vi "Configure Edge Trigger.vi"(6 "HF Rejection":bool=TRUE, 7 "Level":dbl, 8 "error in (no error)":errorcluster, 9 "Slope":u16(ring) items=["Rising", "Falling"], 10 "Function":u16(ring) items=["Voltage: DC", "Voltage: AC", "Current: DC", "Current: AC", "2W Resistance", "4W Resistance", "Diode", "Capacitance", "Temperature", "Continuity", "Frequency", "Period", "Ratio", "Digitize Voltage", "Digitize Current"], 11 "VISA resource name":refnum<visa-resource-name>) -> (0 "error out":errorcluster, 3 "VISA resource name out":refnum<visa-resource-name>)   [LabVIEW 2021, in "Keithley DMM7510.lvlib"]
doc: "This VI sets the slope and level of the analog edge trigger. This also enables or disables the high frequency rejection for analog trigger."
uses:
  Keithley DMM7510.lvlib
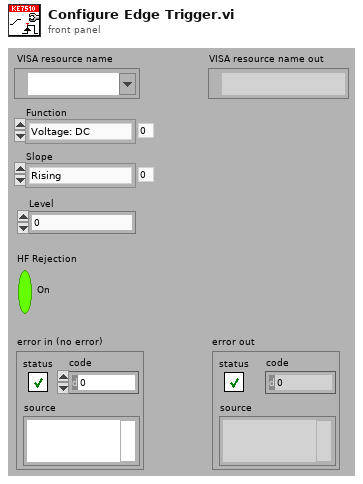
[diagram p1: front panel]
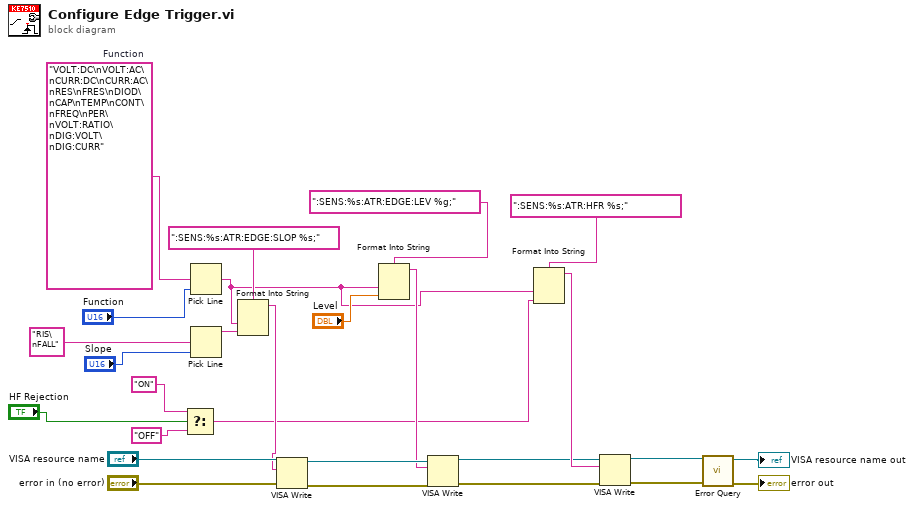
[diagram p0: block diagram]
diagram:
  w23 = "VOLT:DC\nVOLT:AC\nCURR:DC\nCURR:AC\nRES\nFRES\nDIOD\nCAP\nTEMP\nCONT\nFREQ\nPER\nVOLT:RATIO\nDIG:VOLT\nDIG:CURR"  # Function
  n1 = Select(t="ON" ("format string"), s="HF Rejection", f="OFF" ("format string")) -> (s? t:f=w2:string)
  n2 = Pick Line(multi-line string=w23, line index="Function") -> (output string=w8:string)  [unwired: 1 in]
  n3 = Pick Line(multi-line string="RIS\nFALL", line index="Slope") -> (output string=w21:string)  [unwired: 1 in]
  n4 = Format Into String(format string=":SENS:%s:ATR:EDGE:SLOP %s;", w8, w21) -> (resulting string=w15:string)  [unwired: 2 in, 1 out]
  n5 = VISA Write(VISA resource name="VISA resource name", write buffer=w15, error in (no error)="error in (no error)") -> (VISA resource name out=w14:refnum<visa-resource-name>, error out=w13:errorcluster)  [unwired: 1 out]
  n6 = Format Into String(format string=":SENS:%s:ATR:EDGE:LEV %g;", w8, "Level") -> (resulting string=w12:string)  [unwired: 2 in, 1 out]
  n7 = VISA Write(VISA resource name=w14, write buffer=w12, error in (no error)=w13) -> (VISA resource name out=w6:refnum<visa-resource-name>, error out=w3:errorcluster)  [unwired: 1 out]
  n8 = Format Into String(format string=":SENS:%s:ATR:HFR %s;", w8, w2) -> (resulting string=w7:string)  [unwired: 2 in, 1 out]
  n9 = VISA Write(VISA resource name=w6, write buffer=w7, error in (no error)=w3) -> (VISA resource name out=w5:refnum<visa-resource-name>, error out=w4:errorcluster)  [unwired: 1 out]
  n10 = call "Error Query.vi"("error in (no error)"=w4, "VISA resource name"=w5) -> ("error out"=→"error out":errorcluster, "VISA resource name out"=→"VISA resource name out":refnum<visa-resource-name>)  [unwired: 6 in, 2 out]
